vi "fix all paths.vi"(11 "paths":T2) -> (1 "settings":T1, 2 "found":bool[](array[boolean]), 3 "paths out":path[](array[path]))   [LabVIEW 2019]
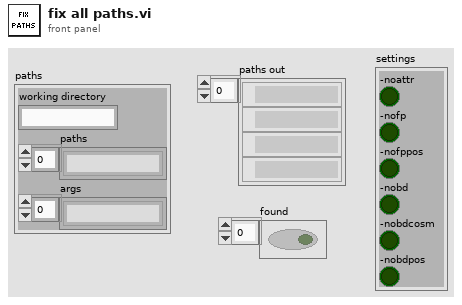
[diagram p1: front panel]
types:
  T1 = cluster{"-noattr":bool, "-nofp":bool, "-nofppos":bool, "-nobd":bool, "-nobdcosm":bool, "-nobdpos":bool}
  T2 = cluster{"working directory":string, "paths":string[], "args":string[]}
  T3 = cluster{"[0]":bool, "[1]":bool, "[2]":bool, "[3]":bool, "[4]":bool, "[5]":bool}
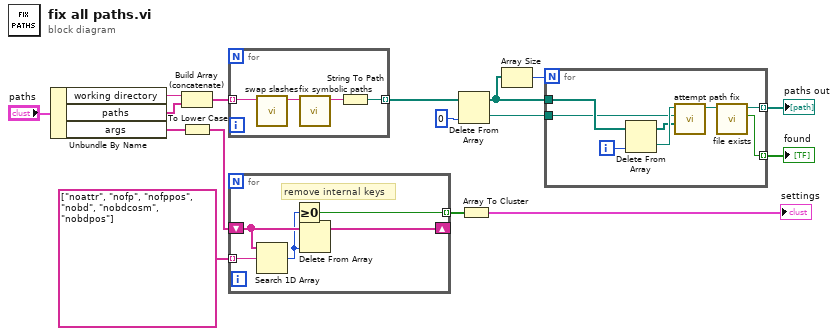
[diagram p0: block diagram]
diagram:
  n1 = Unbundle By Name("paths") -> ("working directory"=w7:string, "paths"=w8:string[], "args"=w5:string[])
  n2 = Build Array (concatenate)(w7, w8) -> (w6:string[])
  n3 = To Lower Case(string=w5) -> (all lower case string=w4:string[])
  n4 = for {
    tunnel: [w18] -> w10 mode=indexing
    tunnel: w6 -> [w17] mode=indexing
    n5 = call "swap slashes.vi"("in"=w17) -> ("out"=w20:string)  [unwired: 10 in]
    n6 = call "fix symbolic paths.vi"("in"=w20) -> ("out"=w19:string)  [unwired: 10 in]
    n7 = String To Path(string=w19) -> (path=w18:path)
  }
  n8 = for {
    shift-right: [w23] -> _
    shift-left: w4 -> [w24]
    tunnel: string[] ["noattr", "nofp", "nofppos", "nobd", "nobdcosm", "nobdpos"] ("lv version keys") -> [w25] mode=indexing
    tunnel: [w21] -> w2 mode=indexing
    # "remove internal keys"
    n9 = Search 1D Array(1D array=w24, element=w25) -> (index of element=w22:i32)  [unwired: 1 in]
    n10 = Greater Or Equal To 0?(x=w22) -> (x >= 0?=w21:bool)
    n11 = Delete From Array(array=w24, index=w22) -> (array with subset deleted=w23:string[])  [unwired: 1 in, 1 out]
  }
  n12 = Delete From Array(array=w10, index=0) -> (deleted portion=w11:path, array with subset deleted=w15:path[])  [unwired: 1 in]
  n13 = Array To Cluster(array=w2) -> (cluster=→"settings":T3)
  n14 = Array Size(array=w15) -> (size(s)=w14:i32)
  n15 = for {
    N: w14 -> [_]
    tunnel: w15 -> [w33]
    tunnel: w11 -> [w29]
    tunnel: [w27] -> w12 mode=indexing
    tunnel: [w26] -> w13 mode=indexing
    i -> [w32]
    n16 = Delete From Array(array=w33, index=w32) -> (deleted portion=w31:path, array with subset deleted=w30:path[])  [unwired: 1 in]
    n17 = call "attempt path fix.vi"("other possible paths"=w30, "working directory"=w29, "path to fix"=w31) -> ("path out"=w28:path)  [unwired: 8 in]
    n18 = call "file exists.vi"("Path in"=w28) -> ("file exists"=w26:bool, "Path out"=w27:path)  [unwired: 9 in]
  }
  "found" <- w13
  "paths out" <- w12
